vi "Encoders.vi"(3 "Reset All":bool) -> (0 "Avg Absolute Rate":dbl, 1 "Avg Absolute Distance":dbl)   [LabVIEW 2017]
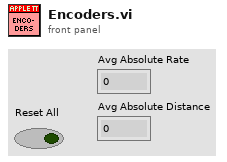
[diagram p1: front panel]
types:
  T1 = typedef "WPI_EncoderDevRef.ctl" = cluster{"DevStatus":errorcluster, "EncoderIndex":T2, "CounterIndex":T3, "DistancePerCount":dbl, "Decoding Type":T4}
  T2 = typedef "FPGA_EncoderIdx.ctl" = enum8{"Enc 0", "Enc 1", "Enc 2", "Enc 3", "Enc 4", "Enc 5", "Enc 6", "Enc 7", "Invalid"}
  T3 = typedef "FPGA_CounterCtrSystemIndex.ctl" = enum8{"Ctr 0", "Ctr 1", "Ctr 2", "Ctr 3", "Ctr 4", "Ctr 5", "Ctr 6", "Ctr 7", "Invalid"}
  T4 = typedef "WPI_EncoderType.ctl" = enum16{"1x", "2x", "4x"}
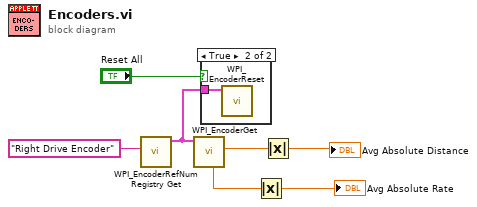
[diagram p0: block diagram]
diagram:
  n1 = call <vilib>:"WPI_EncoderRefNum Registry Get.vi"("refnum name"="Right Drive Encoder") -> ("EncoderDevRef"=w5:T1)  [unwired: 9 in, 1 out]
  n2 = call <vilib>:"WPI_EncoderGet.vi"("EncoderDevRef"=w5) -> ("Distance"=w3:dbl, "Rate"=w4:dbl)  [unwired: 5 in, 4 out]
  n3 = case shown="True" "Reset All" {
    tunnel: w5 -> [_ w8]
    frame False {
    }
    frame True {
      n4 = call <vilib>:"WPI_EncoderReset.vi"("EncoderDevRef"=w8) -> ()  [unwired: 9 in, 2 out]
    }
  }
  n5 = Absolute Value(x=w4) -> (abs(x)=→"Avg Absolute Rate":dbl)
  n6 = Absolute Value(x=w3) -> (abs(x)=→"Avg Absolute Distance":dbl)
